vi "Queue-Modify Time Entry.vi"(8 "error in":errorcluster, 10 "Data":variant, 11 "Queue In":refnum<queue>) -> (0 "error out":errorcluster, 3 "Queue Out":refnum<queue>)   [LabVIEW 2020, in "Main_Process.lvlib" / "Internal Messaging Library.lvlib"]
doc: "<B>Description:</B> Sends Data to the Modify Time Entry Case of Internal Processing for the Event Logger.\n\n<B>Date:</B> 10/2019 \n<B>Author:</B> Choose Movement Consulting, LLC"
uses:
  Internal Messaging Library.lvlib
  Controls/Messaging Cluster.ctl
  Controls/Message.ctl
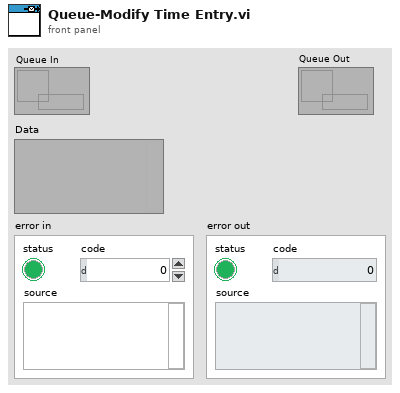
[diagram p1: front panel]
types:
  T1 = typedef "Main_Process.lvlib/Internal Messaging Library.lvlib/Message.ctl" = enum16{"Initialize", "Exit", "Error", "Load Data", "Add Time Entry", "Modify Time Entry", "Delete Time Entry"}
  T2 = typedef "Main_Process.lvlib/Internal Messaging Library.lvlib/Messaging Cluster.ctl" = cluster{"Message":T1, "Data":variant}
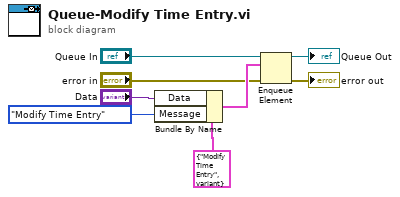
[diagram p0: block diagram]
diagram:
  n1 = Bundle By Name(cluster=T2 {"Message"=enum."Modify Time Entry", "Data"=variant} ("Messaging Cluster"), "Data"="Data", "Message"=Message."Modify Time Entry") -> (w8:T2)
  n2 = Enqueue Element(queue="Queue In", element=w8, error in (no error)="error in") -> (queue out=→"Queue Out":refnum<queue>, error out=→"error out":errorcluster)  [unwired: 1 in, 1 out]
